vi "Sequence Control.vi"(8 "error in (no error)":errorcluster, 11 "Sequencer Module runtime in":refnum<class "Sequencer Module runtime.lvclass">) -> (0 "error out":errorcluster, 3 "Sequencer Module runtime out":refnum<class "Sequencer Module runtime.lvclass">)   [LabVIEW 2015, in "Sequencer Module runtime.lvclass"]
uses:
  Sequencer Module runtime.lvclass
  Sequencer Module runtime.lvclass/Sequencer Module runtime.ctl
  classes/Sequence/Sequence.lvclass
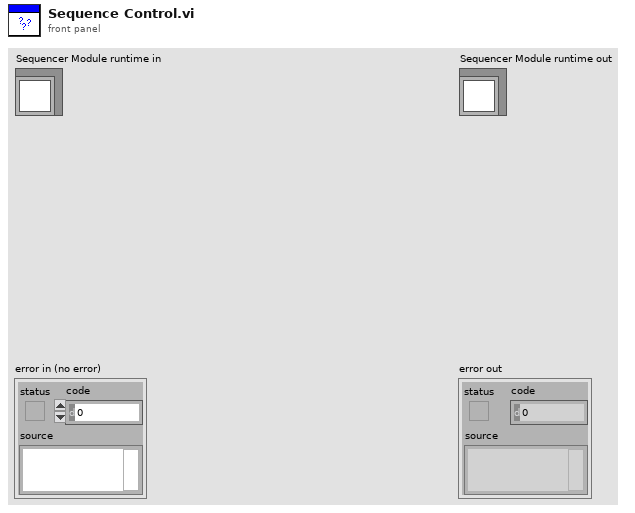
[diagram p1: front panel]
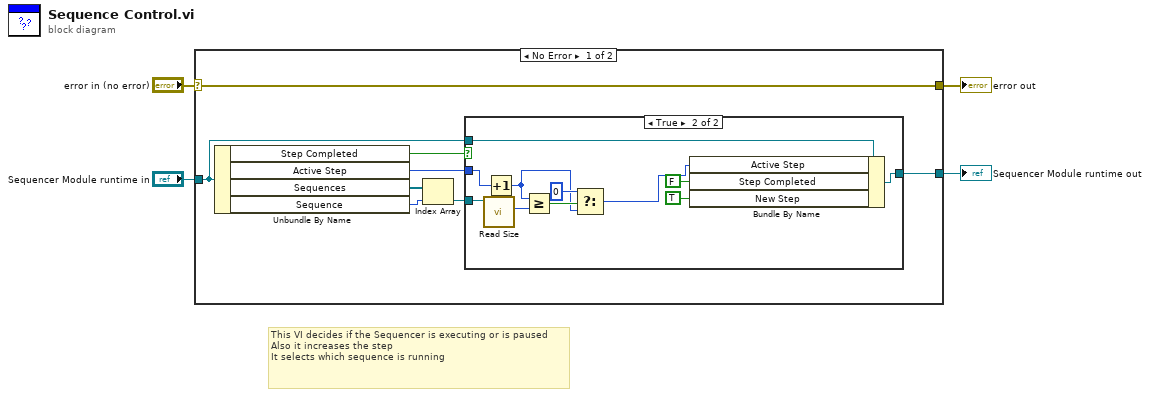
[diagram p0: block diagram]
diagram:
  # "This VI decides if the Sequencer is executing or is paused\nAlso it increases the step \nIt selects which sequence is running"
  n1 = case shown="No Error" "error in (no error)" {
    selector: "error in (no error)" -> [w12 w26]
    tunnel: [w12 w26] -> w3
    tunnel: [w10 w25] -> w1
    tunnel: "Sequencer Module runtime in" -> [w11 w25]
    frame No Error {
      n2 = Unbundle By Name(w11) -> ("Step Completed"=w9:bool, "Active Step"=w5:i32, "Sequences"=w8:refnum<class "Sequence.lvclass">[], "Sequence"=w7:i32)
      n3 = Index Array(array=w8, index=w7) -> (element=w6:refnum<class "Sequence.lvclass">)
      n4 = case shown="True" w9 {
        tunnel: w11 -> [w13 w24]
        tunnel: [w13 w23] -> w10
        tunnel: w6 -> [_ w22]
        tunnel: w5 -> [_ w16]
        frame False {
        }
        frame True {
          n5 = call "Read Size.vi"("Sequence in"=w22) -> ("Size"=w21:i32)  [unwired: 8 in, 2 out]
          n6 = Increment(x=w16) -> (x+1=w15:i32)
          n7 = Greater Or Equal?(x=w15, y=w21) -> (x >= y?=w18:bool)
          n8 = Select(t=0, s=w18, f=w15) -> (s? t:f=w14:i32)
          n9 = Bundle By Name(cluster=w24, "Active Step"=w14, "Step Completed"=FALSE ("Sequencer State.Step Completed"), "New Step"=TRUE ("Sequencer State.New Step")) -> (w23:refnum<class "Sequencer Module runtime.lvclass">)
        }
      }
    }
    frame Error {
    }
  }
  "error out" <- w3
  "Sequencer Module runtime out" <- w1
